vi "Create Network Stream Initiator.vi"(6 "Buffer Size":i32=4096, 7 "Local Address":string, 8 "Remote Context":string, 9 "Remote Name":string, 10 "Remote Address":string, 11 "Name":string) -> (3 "Network Stream Initiator out":refnum<class "Network Stream Initiator.lvclass">)   [LabVIEW 2023, in "Network Stream Initiator.lvclass"]
doc: "Use this method to configure a Network Stream Initiator with connection information for its remote counterpart."
uses:
  Network Stream Initiator.lvclass
  D:/gitlab/network-endpoint-actors/vi.lib/ni/Actors/Network Endpoint Actors/Protocols/Network Stream Strategy/Network Stream/Network Stream.lvclass
  Network Stream/Network Stream.lvclass/Network Stream.ctl
  Network Stream Initiator.lvclass/Network Stream Initiator.ctl
  Network Stream/Network Stream.lvclass
  C:/Program Files/National Instruments/LabVIEW 2023/vi.lib/ni/Actors/Network Endpoint Actors/Abstract Classes/Message Stream/Message Stream.lvclass
  D:/gitlab/network-endpoint-actors/vi.lib/ni/Actors/Network Endpoint Actors/Protocols/Network Stream Strategy/Network Stream Initiator/Network Stream Initiator.lvclass
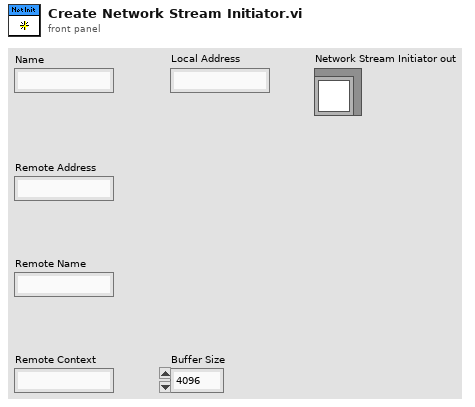
[diagram p1: front panel]
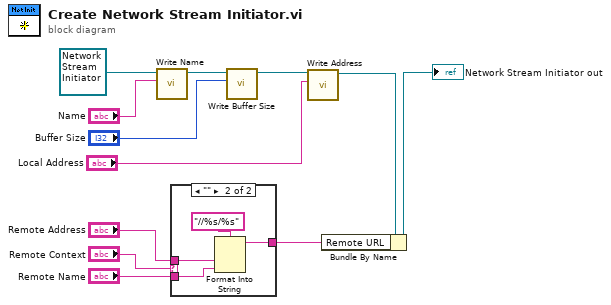
[diagram p0: block diagram]
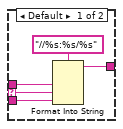
[diagram p2: hidden frame]
diagram:
  n1 = call "Write Name.vi"("Name"="Name", "Network Stream in"=refnum<class "Network Stream Initiator.lvclass"> refnum ("Network Stream Initiator in")) -> ("Network Stream out"=w6:refnum<class "Network Stream Initiator.lvclass">)  [unwired: 9 in]
  n2 = case shown="\"\"" "Remote Context" {
    selector: "Remote Context" -> [w14 _]
    tunnel: [w16 w20] -> w8
    tunnel: "Remote Name" -> [w15 w19]
    tunnel: "Remote Address" -> [w13 w18]
    frame Default {
      n3 = Format Into String(format string="//%s:%s/%s", w13, w14, w15) -> (resulting string=w16:string)  [unwired: 2 in, 1 out]
    }
    frame "" {
      n4 = Format Into String(format string="//%s/%s", w18, w19) -> (resulting string=w20:string)  [unwired: 2 in, 1 out]
    }
  }
  n5 = call "Write Buffer Size.vi"("Buffer Size"="Buffer Size", "Network Stream in"=w6) -> ("Network Stream out"=w3:refnum<class "Network Stream Initiator.lvclass">)  [unwired: 9 in]
  n6 = call "Write Address.vi"("Address"="Local Address", "Network Stream"=w3) -> ("Network Stream out"=w2:refnum<class "Network Stream Initiator.lvclass">)  [unwired: 9 in]
  n7 = Bundle By Name(cluster=w2, "Remote URL"=w8) -> (→"Network Stream Initiator out":refnum<class "Network Stream Initiator.lvclass">)
